vi "Entry.vi"(8 "error in (no error)":errorcluster, 11 "New State":refnum<class "Cursor.lvclass">) -> (0 "error out":errorcluster, 3 "State out":refnum<class "Cursor.lvclass">)   [LabVIEW 2020, in "Keypad.lvlib" / "Cursor.lvclass"]
doc: "This is an abstract method. Override this method to define the behavior when you enter the state."
uses:
  Cursor.lvclass
  Keypad/Keypad.lvclass
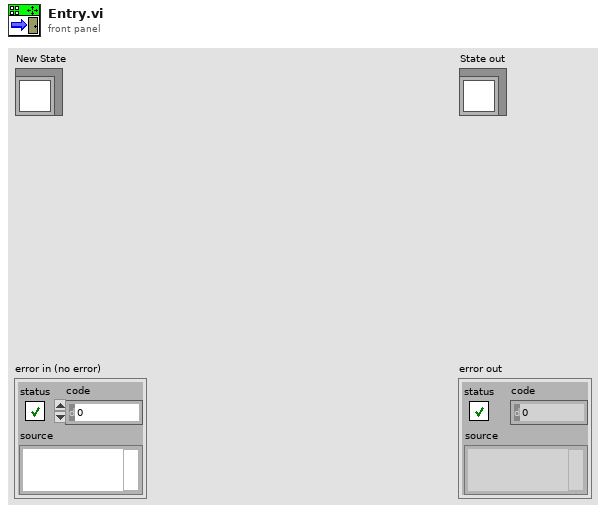
[diagram p1: front panel]
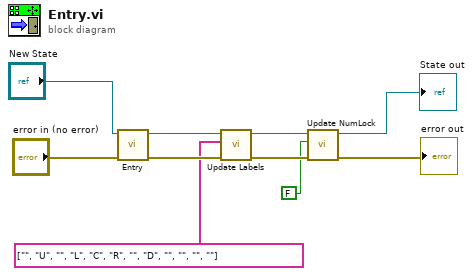
[diagram p0: block diagram]
diagram:
  n1 = call-parent "Entry.vi"("error in (no error)"="error in (no error)", "New State"="New State") -> ("error out"=w8:errorcluster, "State out"=w7:refnum<class "Cursor.lvclass">)  [unwired: 8 in]
  n2 = call "Update Labels.vi"("error in (no error)"=w8, "Labels"=string[] ["", "U", "", "L", "C", "R", "", "D", "", "", "", ""], "Keypad in"=w7) -> ("error out"=w4:errorcluster, "Keypad out"=w5:refnum<class "Cursor.lvclass">)  [unwired: 7 in]
  n3 = call "Update NumLock.vi"("error in (no error)"=w4, "NuLockS State"=FALSE, "Keypad in"=w5) -> ("error out"=→"error out":errorcluster, "Keypad out"=→"State out":refnum<class "Cursor.lvclass">)  [unwired: 7 in]
